vi "Init Tree Control.vi"(8 "error in (no error)":errorcluster, 11 "TreeControl in":refnum<vi>) -> (0 "error out":errorcluster, 3 "TreeControl out":refnum<vi>)   [LabVIEW 2026, in "VILab.lvlib"]
uses:
  VILab.lvlib
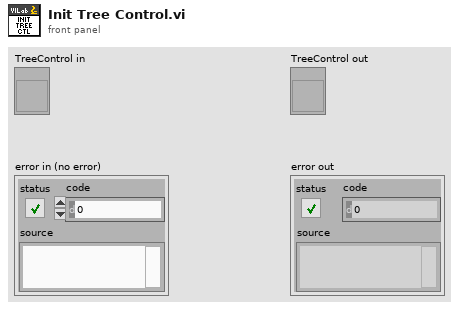
[diagram p1: front panel]
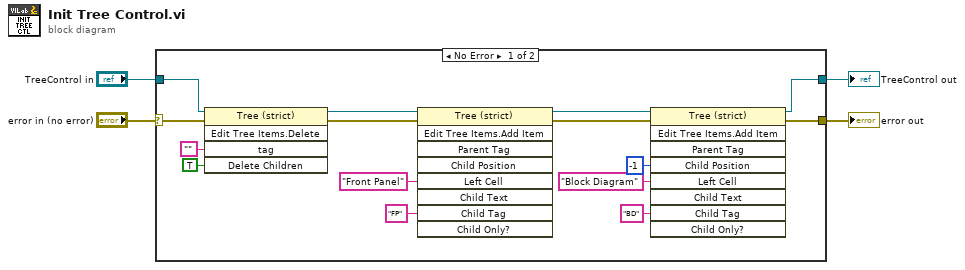
[diagram p0: block diagram]
diagram:
  n1 = case shown="No Error" "error in (no error)" {
    selector: "error in (no error)" -> [w8 w20]
    tunnel: "TreeControl in" -> [w5 w21]
    tunnel: [w10 w20] -> w2
    tunnel: [w9 w21] -> w1
    frame No Error {
      n2 = invoke class="Tree (strict)" method="Edit Tree Items.Delete"(reference=w5, error in=w8, "tag"="" ("Tag"), "Delete Children"=TRUE ("Delete Children?")) -> (reference out=w6:refnum<vi>, error out=w7:errorcluster)  [unwired: 1 in, 3 out]
      n3 = invoke class="Tree (strict)" method="Edit Tree Items.Add Item"(reference=w6, error in=w7, "Left Cell"="Front Panel" ("Left Cell String"), "Child Tag"="FP") -> (reference out=w16:refnum<vi>, error out=w11:errorcluster)  [unwired: 5 in, 7 out]
      n4 = invoke class="Tree (strict)" method="Edit Tree Items.Add Item"(reference=w16, error in=w11, "Child Position"=-1, "Left Cell"="Block Diagram" ("Left Cell String"), "Child Tag"="BD") -> (reference out=w9:refnum<vi>, error out=w10:errorcluster)  [unwired: 4 in, 7 out]
    }
    frame Error {
    }
  }
  "error out" <- w2
  "TreeControl out" <- w1
